vi "getfracLUT.vi"() -> ()   [LabVIEW 2012]
panel:
  out "Init Data Out":u16[](array[numeric])
  in  "Frequency":dbl=1000.0
  in  "Number of entries in LUT":dbl=512.0
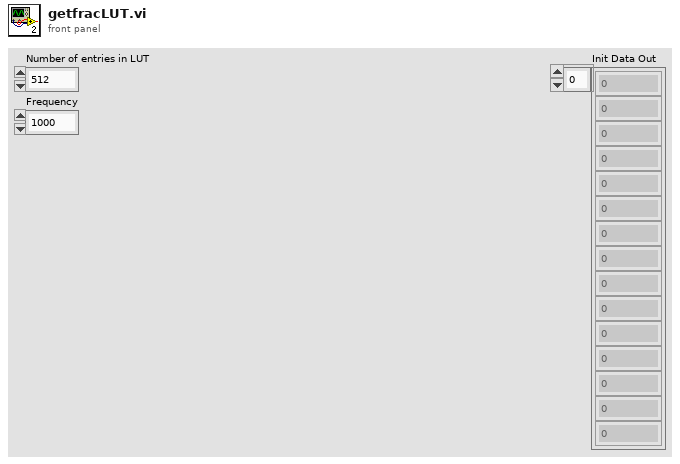
[diagram p1: front panel]
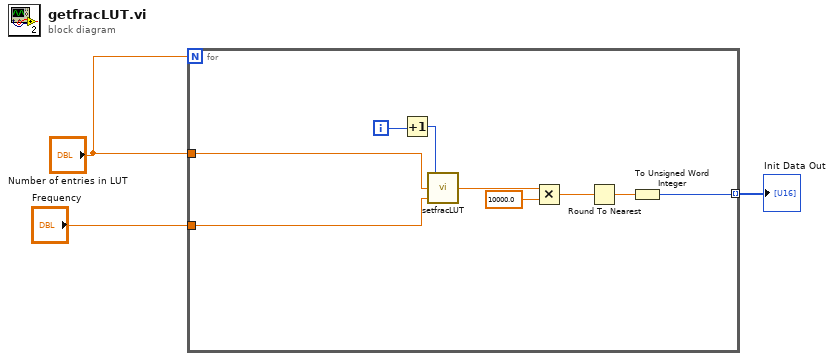
[diagram p0: block diagram]
diagram:
  n1 = for {
    N: "Number of entries in LUT" -> [_]
    tunnel: "Number of entries in LUT" -> [w12]
    tunnel: "Frequency" -> [w9]
    tunnel: [w4] -> w1 mode=indexing
    i -> [w11]
    n2 = Increment(x=w11) -> (x+1=w10:i32)
    n3 = call "setfracLUT.vi"("Frequency"=w9, "Number of entries in LUT"=w12, "Input"=w10) -> ("Fraction"=w8:dbl)
    n4 = Multiply(x=w8, y=10000.0) -> (x*y=w6:dbl)
    n5 = Round To Nearest(number=w6) -> (nearest integer value=w5:dbl)
    n6 = To Unsigned Word Integer(number=w5) -> (unsigned 16bit integer=w4:u16)
  }
  "Init Data Out" <- w1
